vi "Variable@Publish__Parameter.vi"(1 "ParamterIn":string) -> (0 "ParamterOut":string)   [LabVIEW 2020]
panel:
  in  "ParameterName":string(combo)
  in  "Confirm":bool
  # "Variable@Publish $Variable1(,$Variable2,$Variable3......)"
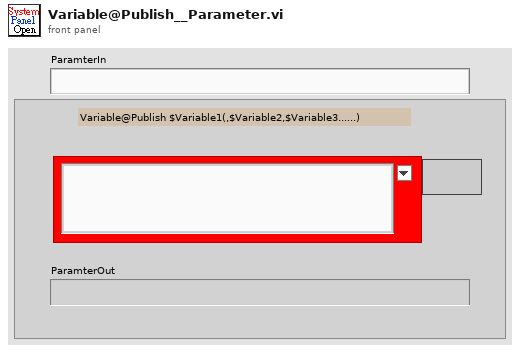
[diagram p1: front panel]
types:
  T1 = enum16{"Get", "Init", "Set", "Delete", "GetElement", "Inc", "Dec", "ReName"}
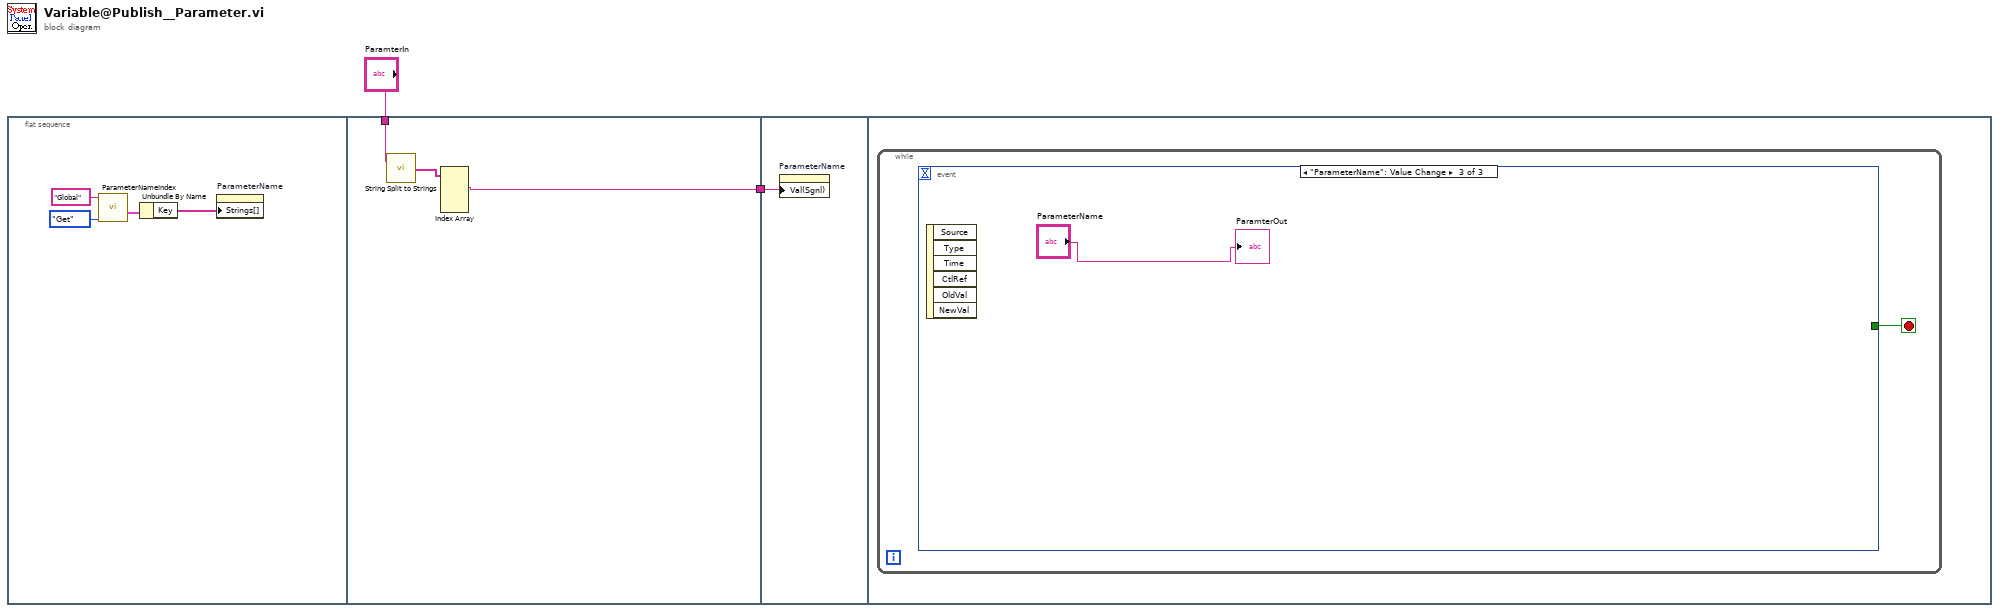
[diagram p0: block diagram]
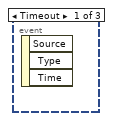
[diagram p2: hidden frame]
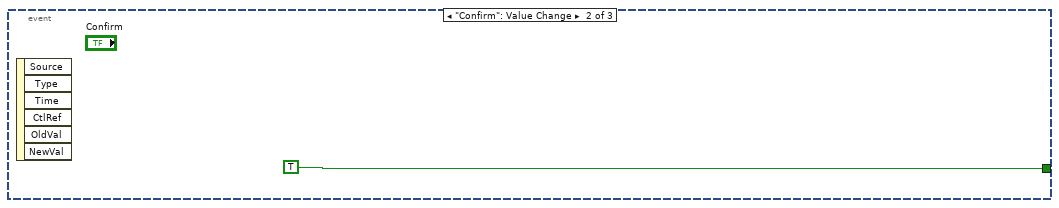
[diagram p3: hidden frame]
diagram:
  n1 = flat-sequence {
    tunnel: "ParamterIn" -> [w9]
    tunnel: [w7] -> w1
    tunnel: w1 -> [w10]
    frame #0 {
      n2 = call "ParameterNameIndex.vi"("OP"=T1."Get", "VariableSection"="Global") -> ("GlobalKeyValue"=w6:cluster{"Key":string[], "Value":string[]})  [unwired: 3 in, 6 out]
      n3 = Unbundle By Name(w6) -> ("Key"=w5:string[])
      n4 = property on="ParameterName" class="CmbBox"("Strings[]"=w5) -> ()  [unwired: 2 in, 2 out]
    }
    frame #1 {
      n5 = call "String Split to Strings.vi"("String"=w9) -> ("Array"=w8:string[])  [unwired: 1 in]
      n6 = Index Array(array=w8) -> (element #1=w7:string)  [unwired: 4 in, 3 out]
    }
    frame #2 {
      n7 = property on="ParameterName" class="CmbBox"("Val(Sgnl)"=w10) -> ()  [unwired: 2 in, 2 out]
    }
    frame #3 {
      n8 = while {
        stop <- w11 stop-if-true
        n9 = event shown="[2] \"ParameterName\": Value Change" {
          selector: _ -> [_ _ _]
          dyn-events: _ -> [_ _ _]
          timeout: _ -> [_ _ _]
          tunnel: [_ TRUE _] -> w11
          event Timeout {
            n10 = event-data() -> ()  [unwired: 1 in, 3 out]
          }
          event "Confirm": Value Change {
            n11 = event-data() -> ()  [unwired: 1 in, 6 out]
          }
          event "ParameterName": Value Change {
            n12 = event-data() -> ()  [unwired: 1 in, 6 out]
            "ParamterOut" <- "ParameterName"
          }
        }
      }
    }
  }
